vi "WSP2_PartNumberRef.vi"(2 "BCTYPE":i8, 3 "SerialNumber":string) -> (0 "error out":errorcluster, 1 "AssemblyPartNumber":string)   [LabVIEW 2022 SP3]
uses:
  C:/Elatch-Bench-Test/WSConnector/WSConnector.dll
  WSConnector/WSConnector.dll
panel:
  out "Cimp_AssemblyPartNumber":string
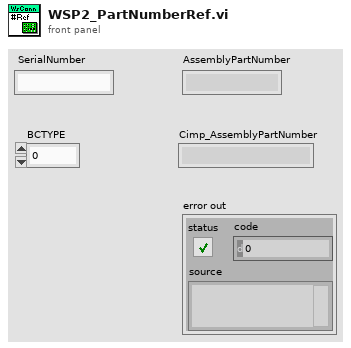
[diagram p1: front panel]
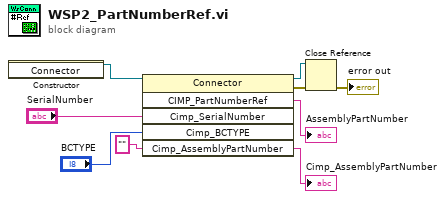
[diagram p0: block diagram]
diagram:
  n1 = constructor class="Connector"() -> (reference out=w9:refnum<k24>)  [unwired: 3 in, 2 out]
  n2 = invoke class="Connector" method="CIMP_PartNumberRef"(reference=w9, "Cimp_SerialNumber"="SerialNumber", "Cimp_BCTYPE"="BCTYPE", "Cimp_AssemblyPartNumber"="") -> (reference out=w1:refnum<k24>, error out=w2:errorcluster, "CIMP_PartNumberRef"=→"AssemblyPartNumber":string, "Cimp_AssemblyPartNumber"=→"Cimp_AssemblyPartNumber":string)  [unwired: 2 in, 2 out]
  n3 = Close Reference(reference=w1, error in (no error)=w2) -> (error out=→"error out":errorcluster)
